vi "SQLite Add Balance Test.vi"(7 "Test DB Set Up Command":string, 8 "Error In (no error)":errorcluster, 11 "SQLite DB Operator In":refnum<class "SQLite DB Operator.lvclass">) -> (0 "Error Out":errorcluster, 3 "SQLite DB Operator Out":refnum<class "SQLite DB Operator.lvclass">)   [LabVIEW 2023]
uses:
  Clasess/SQLite DB Operator/SQLite DB Operator.lvclass
  Clasess/DB Records/Expenses Tracker Balance/Public/Ctrls/Balance.ctl
  Clasess/DB Records/Expenses Tracker Balance/Expenses Tracker Balance.lvclass
  H:/Desktop/LabVIEW/LabView Repo/Expenses-Tracker-DB-Operator/Interfaces/Expenses Tracker Record/Expenses Tracker Record.lvclass
  <vilib>/drjdpowell/SQLite Library/SQL Connection/Execute SQL (1D Cluster).vi
  <vilib>/addons/_JKI Toolkits/Caraya/classes/Assert/Assert Equal Value_Variant.vi
  <vilib>/addons/_JKI Toolkits/Caraya/classes/Test/Test.lvclass
  <vilib>/addons/_JKI Toolkits/Caraya/classes/Assert/Assert.lvclass
  <vilib>/drjdpowell/SQLite Library/SQLite.lvlib
  <vilib>/drjdpowell/SQLite Library/SQL Connection/Connection.lvclass
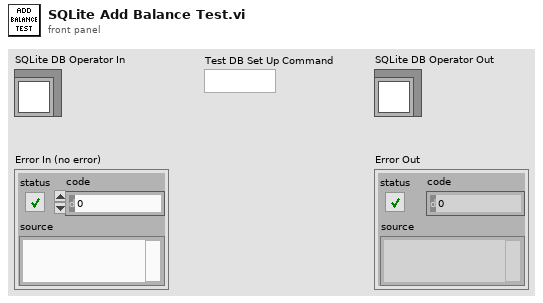
[diagram p1: front panel]
types:
  T1 = typedef "Expenses Tracker Balance.lvclass/Balance.ctl" = cluster{"ID":u8, "Value":dbl, "Last_update":timestamp}
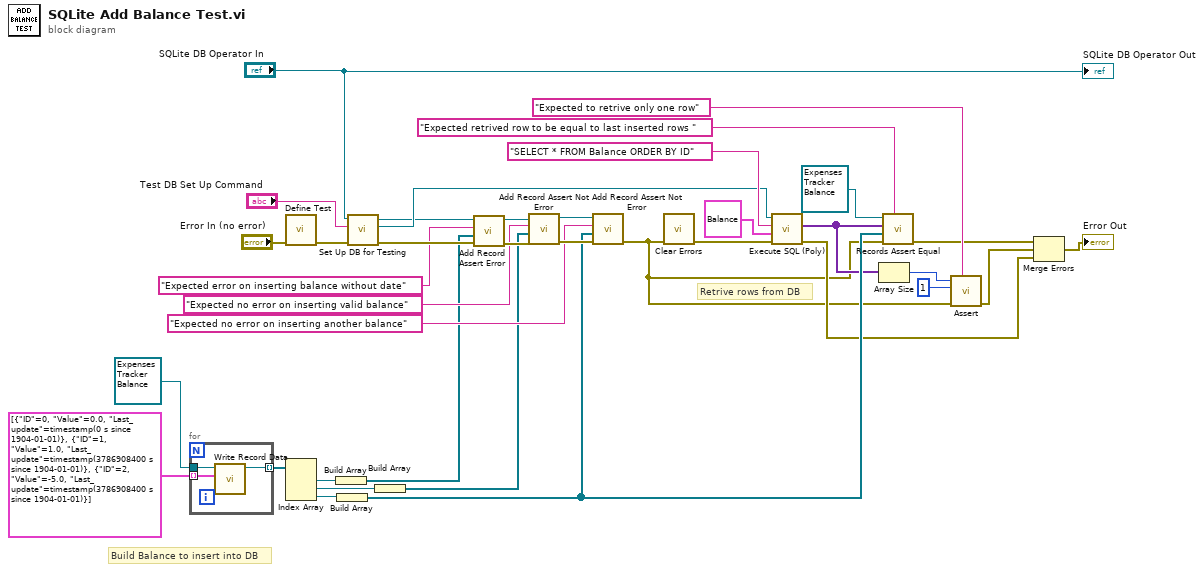
[diagram p0: block diagram]
diagram:
  # "Retrive rows from DB"
  # "Build Balance to insert into DB"
  n1 = for {
    tunnel: T1[] [{"ID"=0, "Value"=0.0, "Last_update"=timestamp(0 s since 1904-01-01)}, {"ID"=1, "Value"=1.0, "Last_update"=timestamp(3786908400 s since 1904-01-01)}, {"ID"=2, "Value"=-5.0, "Last_update"=timestamp(3786908400 s since 1904-01-01)}] ("Array") -> [w40] mode=indexing
    tunnel: refnum<class "Expenses Tracker Balance.lvclass"> refnum ("Expenses Tracker Category") -> [w39]
    tunnel: [w38] -> w34 mode=indexing
    n2 = call-dynamic "Write Record Data.vi"("Record"=w40, "Expenses Tracker Balance In"=w39) -> ("Expenses Tracker Balance Out"=w38:refnum<class "Expenses Tracker Balance.lvclass">)  [unwired: 8 in, 1 out]
  }
  n3 = call <vilib>:"Define Test.vi"("error in (no error)"="Error In (no error)") -> ("error out"=w24:errorcluster)  [unwired: 9 in, 1 out]
  n4 = Index Array(array=w34) -> (element #1=w33:refnum<class "Expenses Tracker Balance.lvclass">, element #2=w32:refnum<class "Expenses Tracker Balance.lvclass">, element #3=w29:refnum<class "Expenses Tracker Balance.lvclass">)  [unwired: 3 in]
  n5 = Build Array(w33) -> (w10:refnum<class "Expenses Tracker Balance.lvclass">[])
  n6 = Build Array(w29) -> (w8:refnum<class "Expenses Tracker Balance.lvclass">[])
  n7 = call "Set Up DB for Testing.vi"("Error In (no error)"=w24, "Test DB Set Up Command"="Test DB Set Up Command", "SQLite DB Operator In"="SQLite DB Operator In") -> ("Error Out"=w18:errorcluster, "SQLite Connection"=w23:refnum<class "Connection.lvclass">, "SQLite DB Operator Out"=w14:refnum<class "SQLite DB Operator.lvclass">)  [unwired: 6 in]
  n8 = Build Array(w32) -> (w9:refnum<class "Expenses Tracker Balance.lvclass">[])
  n9 = call "Add Record Assert Error.vi"("Error In"=w18, "Records"=w10, "Assertion Label"="Expected error on inserting balance without date" ("Label (VI Title)"), "SQLite DB Operator In"=w14) -> ("Error Out"=w21:errorcluster, "SQLite DB Operator Out"=w22:refnum<class "SQLite DB Operator.lvclass">)  [unwired: 6 in]
  n10 = call "Add Record Assert Not Error.vi"("Error In"=w21, "Records"=w9, "Assertion Label"="Expected no error on inserting valid balance" ("Label (VI Title)"), "SQLite DB Operator In"=w22) -> ("Error Out"=w19:errorcluster, "SQLite DB Operator Out"=w20:refnum<class "SQLite DB Operator.lvclass">)  [unwired: 6 in]
  n11 = call "Add Record Assert Not Error.vi"("Error In"=w19, "Records"=w8, "Assertion Label"="Expected no error on inserting another balance" ("Label (VI Title)"), "SQLite DB Operator In"=w20) -> ("Error Out"=w1:errorcluster)  [unwired: 6 in, 1 out]
  n12 = call <vilib>:"Clear Errors.vi"("error in (no error)"=w1) -> ("error out"=w6:errorcluster)  [unwired: 5 in, 1 out]
  n13 = call-poly <vilib>:"Execute SQL (Poly).vi"("error in (no error)"=w6, "Cluster (or Array of Clusters)"=T1 {"ID"=0, "Value"=0.0, "Last_update"=timestamp(0 s since 1904-01-01)} ("Balance"), "SQL"="SELECT * FROM Balance ORDER BY ID", "SQLite Connection in"=w23) -> ("error out"=w2:errorcluster, "Result Set (Array of Clusters)"=w5:variant[])  [unwired: 5 in, 1 out]
  n14 = Array Size(array=w5) -> (size(s)=w28:i32)
  n15 = call "Records Assert Equal.vi"("Assertion Label"="Expected retrived row to be equal to last inserted rows " ("Label (VI Title)"), "Error In"=w1, "Correct Records"=w8, "Typedef Records"=w5, "Expenses Tracker Record In"=refnum<class "Expenses Tracker Balance.lvclass"> refnum ("Expenses Tracker Category")) -> ("Error Out"=w4:errorcluster)  [unwired: 6 in]
  n16 = call-poly <vilib>:"Assert.vi"("Label"="Expected to retrive only one row" ("Label (VI Title)"), "error in (no error)"=w1, "Y"=1, "X"=w28) -> ("error out"=w3:errorcluster)  [unwired: 6 in, 1 out]
  n17 = Merge Errors(w4, w3, w2) -> (→"Error Out":errorcluster)
  "SQLite DB Operator Out" <- "SQLite DB Operator In"
